vi "Save an I32 Image Vector to FITS with Primary and Extension Headers.vi"(4 "FITS info":T4={"File name"="lsob_demo_0530_LM_20190529_124525_live_C1_00020_001_lev0.0.fits", "Date"="2019-05-29T12:45:25"}, 5 "Andor":T1={"Handle"=0, "Pixel Encoding"="", "AOI Width"=0, "AOI Height"=0, "AOI Stride"=0, "Row Readout Time"=0.0, "Frame Readout Time"=0.0, "Interframe Time"=0.0, "Semaphore"=refnum, "SerialNumber"="", "Camera Model"="", "Controller ID"="", "Firmware Version"="", "Shutter"="Global", "BDiv"=1, "Time at Synch"=timestamp(3029526000.379448 s since 1904-01-01), "Idx"=0, "PreAmp"="", "Binning"=enum."1x1", "PixelReadoutRate"="", "Exposure (s)"=0.05, "Image Bytes"=0, "Image Pixels"=0, "SpuriousNoiseFilter"=FALSE, "Overlap"=FALSE, "CycleMode"=""} {"Exposure (s)" format="%^.3g"; "Time at Synch" format="%<%H:%M:%S>T"; "Interframe Time" format="%#_3g"; "Frame Readout Time" format="%_3g"; "Row Readout Time" format="%_3g"}, 6 "byte order (0:big-endian, network order)":T14(ring), 7 "SCD FITS Cluster":T5={"Wavelength (nm)"=530.15, "Exposure (s)"=0.05, "Tuning Delay (ms)"=1000.0, "Beam Type (-1/1)"=1.0, "Tuning Voltages"=[1.111, 2.222, 3.333, 4.444], "Observer"="observer", "Light Shapping Diffuser"=enum."In Beam", "Comment"="", "Data Type"=9, "Mod Cycles"=0, "SCD Calibration Optics"=enum."1 - Polarizer @0, I+Q", "SCD Emission Line Filter"=enum."1-557.6nm", "Cookbook"="", "COMP-S Calibration Wheel"=enum."Dark", "COMP-S Andover Filter Wheel"=enum."530.3nm/HWB 0.34nm (Fe XIV)", "FOV Rotation (deg)"=66.0, "Objective Lens Position (mm)"=0.0, "Occulter size"=0.0, "Time End"=timestamp(3382374145.421875 s since 1904-01-01), "Acc Exposure (s)"=0.0, "Time Stamp Array"=[], "Camera Serial Number"=[], "Camera Temp"=[], "Camera PI (mm)"=[], "Time Start"=timestamp(3382374145.421875 s since 1904-01-01), "Peripherals"={"ILX controler"=FALSE, "Zone temperatures"=FALSE, "Andor"=FALSE, "Andor 2"=FALSE, "PI Stages"=FALSE, "AISAS mechanisms"=FALSE, "AISAS Mech.lvclass"=refnum, "Zone temp ref"=variant, "FWs"=FALSE}, "FITS paths"=[], "Cameras"=enum."Andor", "load preset cbk"=FALSE, "periodic check count"=0} {"Camera PI (mm)" format="%_3g"; "Acc Exposure (s)" format="%^.3g"; "Occulter size" format="%.2f"; "Objective Lens Position (mm)" min=70.0 max=152.0 format="%.2f"; "FOV Rotation (deg)" format="%.1f"; "Data Type" items=["LIVE", "DARK", "FLAT", "CALI", "OBSE", "ABSO", "AURE", "TARG", "OBJE", "HOLE", "OREX", "THRO", "CHIP"]; "Exposure (s)" format="%^.3g"; "Wavelength (nm)" format="%_6g"}, 8 "error in":errorcluster, 9 "Image Data":u32[](array[numeric]), 10 "Image #":i32=1, 11 "FITS File Path":path=path "G:/SCD Data/Level-0/20160930/20160930T203514.fits") -> (0 "error out":errorcluster, 2 "23040 Byte Header":string="SIMPLE  =                              T / CONFORMS TO FITS STANDARD            BITPIX  =                             32 / BITS PER PIXEL                       NAXIS   =                              2 / DATA DIMENSIONS IN FITS FILE         NAXIS1  =                              0 / XDIM (PIXELS)                        NAXIS2  =                              0 / YDIM (PIXELS)                        NAXIS3  =                              4 / 4 POLARIZATION STATES                NAXIS4  =                              1 / 1 CAMERA                             ORIGIN  =                        'AISAS' / SCIENTIFIC GROUP                     OBSERVER=                     'SCHWARTZ' / NAME OF OBSERVER                     TELESCOP=                   '20CM ZEISS' / NAME OF TELESCOPE                    LOCATION=            'LOMNICKY PEAK OBS' / LOCATION OF TELESCOPE                INSTRUME=                          'SCD' / NAME OF INSTRUMENT                   BZERO   =                             0. /  ADU OFFSET                          FOCUS   =                             26 / CAMERA-STAGE POSITION (MM)           ROTPOS  =                           66.0 / ROTATIONAL POSITION (DEG)            DIFFUSER=                      'IN BEAM' / 0=IN BEAM, 1=OUT OF BEAM             FW-WVLNG=                        '557.6' / PRE-FILTER CENTER WAVELENGTH (NM)    FW-CALIB=                         'DARK' / CAL-WHEEL POSITION                   CAM-SN1 =                    'SCC-02209' / CAMERA SERIAL NUMBER                 CAM-TEMP=                       0.000000 / FOCAL PLANE TEMP (C)                 TUNEDLAY=                           1000 / LCVR RELAXATION DELAY (mS)           DATE_OBS=                     '3/7/2011' / DATE OF OBSERVATION START (UTC)      TIME_OBS=                   '212225.421' / TIME OF OBSERVATION (UTC)            EXPOSURE=                       0.050000 / EXPOSURE TIME (S)                    MODC    =                              0 / NUMBER OF IMAGES AT EACH STATE       NLC-1   =                          1.111 / TUNING VOLTAGE-1                     NLC-2   =                          2.222 / TUNING VOLTAGE-2                     NLC-3   =                          3.333 / TUNING VOLTAGE-3                     NLC-4   =                          4.444 / TUNING VOLTAGE-4                     NLC-5   =                          0.000 / TUNING VOLTAGE-5                     BEAM    =                              1 / BEAM (0=ON BAND OR 1=CONTINUUM)      WAVELENG=                         530.15 / WAVELENGTH OF OBS (NM)               COMMHEAD=                             '' / OBSERVER COMMENT                     COOKBOOK=                                / COOKBOOK  LOADED                     COMMENT                                                                         COMMENT                                                                         COMMENT                                                                         COMMENT                                                                         COMMENT                                                                         COMMENT                                                                         COMMENT                                                                         COMMENT                                                                         COMMENT                                                                         COMMENT                                                                         COMMENT                                                                         COMMENT                                                                         COMMENT                                                                         COMMENT                                                                         COMMENT                                                                         COMMENT                                                                         COMMENT                                                                         COMMENT                                                                         COMMENT                                                                         COMMENT                                                                         COMMENT                                                                         COMMENT                                                                         COMMENT                                                                         COMMENT                                                                         COMMENT                                                                         COMMENT                                                                         COMMENT                                                                         COMMENT                                                                         COMMENT                                                                         COMMENT                                                                         COMMENT                                                                         COMMENT                                                                         COMMENT                                                                         COMMENT                                                                         COMMENT                                                                         COMMENT                                                                         COMMENT                                                                         COMMENT                                                                         COMMENT                                                                         COMMENT                                                                         COMMENT                                                                         COMMENT                                                                         COMMENT                                                                         COMMENT                                                                         COMMENT                                                                         COMMENT                                                                         COMMENT                                                                         COMMENT                                                                         COMMENT                                                                         COMMENT                                                                         COMMENT                                                                         COMMENT                                                                         COMMENT                                                                         COMMENT                                                                         COMMENT                                                                         COMMENT                                                                         COMMENT                                                                         COMMENT                                                                         COMMENT                                                                         COMMENT                                                                         COMMENT                                                                         COMMENT                                                                         COMMENT                                                                         COMMENT                                                                         COMMENT                                                                         COMMENT                                                                         COMMENT                                                                         COMMENT                                                                         COMMENT                                                                         COMMENT                                                                         COMMENT                                                                         COMMENT                                                                         COMMENT                                                                         COMMENT                                                                         COMMENT                                                                         COMMENT                                                                         COMMENT                                                                         COMMENT                                                                         COMMENT                                                                         COMMENT                                                                         COMMENT                                                                         COMMENT                                                                         COMMENT                                                                         COMMENT                                                                         COMMENT                                                                         COMMENT                                                                         COMMENT                                                                         COMMENT                                                                         COMMENT                                                                         COMMENT                                                                         COMMENT                                                                         COMMENT                                                                         COMMENT                                                                         COMMENT                                                                         COMMENT                                                                         COMMENT                                                                         COMMENT                                                                         COMMENT                                                                         COMMENT                                                                         COMMENT                                                                         COMMENT                                                                         COMMENT                                                                         COMMENT                                                                         COMMENT                                                                         COMMENT                                                                         COMMENT                                                                         COMMENT                                                                         COMMENT                                                                         COMMENT                                                                         COMMENT                                                                         COMMENT                                                                         COMMENT                                                                         COMMENT                                                                         COMMENT                                                                         COMMENT                                                                         COMMENT                                                                         COMMENT                                                                         COMMENT                                                                         COMMENT                                                                         COMMENT                                                                         COMMENT                                                                         COMMENT                                                                         COMMENT                                                                         COMMENT                                                                         COMMENT                                                                         COMMENT                                                                         COMMENT                                                                         COMMENT                                                                         COMMENT                                                                         COMMENT                                                                         COMMENT                                                                         COMMENT                                                                         COMMENT                                                                         COMMENT                                                                         COMMENT                                                                         COMMENT                                                                         COMMENT                                                                         COMMENT                                                                         COMMENT                                                                         COMMENT                                                                         COMMENT                                                                         COMMENT                                                                         COMMENT                                                                         COMMENT                                                                         COMMENT                                                                         COMMENT                                                                         COMMENT                                                                         COMMENT                                                                         COMMENT                                                                         COMMENT                                                                         COMMENT                                                                         COMMENT                                                                         COMMENT                                                                         COMMENT                                                                         COMMENT                                                                         COMMENT                                                                         COMMENT                                                                         COMMENT                                                                         COMMENT                                                                         COMMENT                                                                         COMMENT                                                                         COMMENT                                                                         COMMENT                                                                         COMMENT                                                                         COMMENT                                                                         COMMENT                                                                         COMMENT                                                                         COMMENT                                                                         COMMENT                                                                         COMMENT                                                                         COMMENT                                                                         COMMENT                                                                         COMMENT                                                                         COMMENT                                                                         COMMENT                                                                         COMMENT                                                                         COMMENT                                                                         COMMENT                                                                         COMMENT                                                                         COMMENT                                                                         COMMENT                                                                         COMMENT                                                                         COMMENT                                                                         COMMENT                                                                         COMMENT                                                                         COMMENT                                                                         COMMENT                                                                         COMMENT                                                                         COMMENT                                                                         COMMENT                                                                         COMMENT                                                                         COMMENT                                                                         COMMENT                                                                         COMMENT                                                                         COMMENT                                                                         COMMENT                                                                         COMMENT                                                                         COMMENT                                                                         COMMENT                                                                         COMMENT                                                                         COMMENT                                                                         COMMENT                                                                         COMMENT                                                                         COMMENT                                                                         COMMENT                                                                         COMMENT                                                                         COMMENT                                                                         COMMENT                                                                         COMMENT                                                                         COMMENT                                                                         COMMENT                                                                         COMMENT                                                                         COMMENT                                                                         COMMENT                                                                         COMMENT                                                                         COMMENT                                                                         COMMENT                                                                         COMMENT                                                                         COMMENT                                                                         COMMENT                                                                         COMMENT                                                                         COMMENT                                                                         COMMENT                                                                         COMMENT                                                                         COMMENT                                                                         COMMENT                                                                         COMMENT                                                                         COMMENT                                                                         COMMENT                                                                         COMMENT                                                                         COMMENT                                                                         COMMENT                                                                         COMMENT                                                                         COMMENT                                                                         COMMENT                                                                         COMMENT                                                                         COMMENT                                                                         COMMENT                                                                         COMMENT                                                                         COMMENT                                                                         COMMENT                                                                         COMMENT                                                                         COMMENT                                                                         COMMENT                                                                         COMMENT                                                                         COMMENT                                                                         COMMENT                                                                         COMMENT                                                                         COMMENT                                                                         COMMENT                                                                         COMMENT                                                                         COMMENT                                                                         COMMENT                                                                         END                                                                             ", 3 "FITS Path Out":path=path "G:/SCD Data/Level-0/20160930/20160930T203514.fits")   [LabVIEW 2014]
doc: "Duplicate first measurement\nand put it in first element of\nmeasurement array. This\nis a dummy measurement for the\nprimary header. This is because\nwe don't want any images associated\nwith the primary HDU, just the \nextensions. In the Make FITS\nHeaders VI, the NAXIS is set to 0 in\nthis primary HDU"
uses:
  Controls/SCD - FITS Cluster.ctl
  AISAS/Mech/AISAS Mech.lvclass
  AISAS/Controls/Diffuser.ctl
  Controls/SCD - Calibration Optics Filter Wheel.ctl
  Controls/SCD - EDT - Emission Line Filter Wheel.ctl
  Controls/CoMP-S Controls/Polarization Optics Filter Wheel.ctl
  Controls/CoMP-S Controls/Emission Line Filter Wheel.ctl
  AISAS/Controls/focus.ctl
  Controls/peripherals.ctl
  Controls/Cameras select.ctl
  Controls/Fits info.ctl
  Camera/Andor Neo Info.ctl
  Controls/beaning.ctl
  Controls/Globals.vi
panel:
  out "NAXIS":string
  out "# Images in Vector":i32=4
  out "Length of Vector":i32=22118400
  out "Total Pixels":i64=5529600
  out "AOI Height":i64=2160
  out "AOI Width":i64=2560
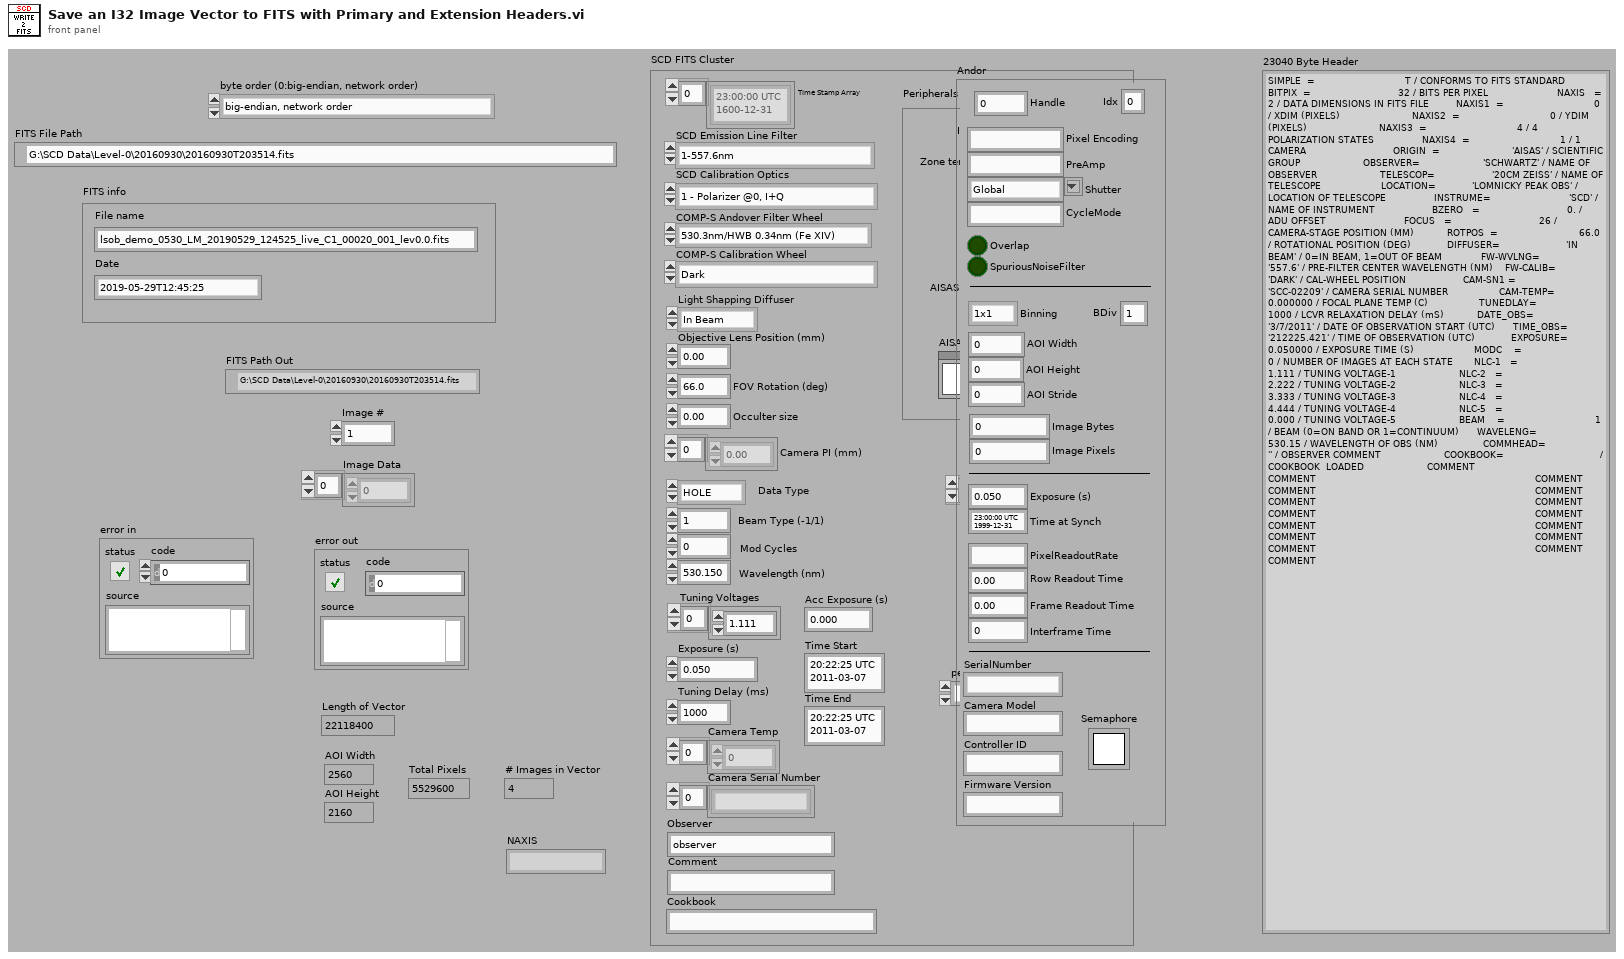
[diagram p1: front panel]
types:
  T1 = typedef "Andor Neo Info.ctl" = cluster{"Handle":i32, "Pixel Encoding":string, "AOI Width":i32, "AOI Height":i32, "AOI Stride":i32, "Row Readout Time":dbl, "Frame Readout Time":dbl, "Interframe Time":dbl, "Semaphore":T2, "SerialNumber":string, "Camera Model":string, "Controller ID":string, "Firmware Version":string, "Shutter":string, "BDiv":u8, "Time at Synch":timestamp, "Idx":i32, "PreAmp":string, "Binning":T3, "PixelReadoutRate":string, "Exposure (s)":dbl, "Image Bytes":i64, "Image Pixels":i64, "SpuriousNoiseFilter":bool, "Overlap":bool, "CycleMode":string}
  T2 = typedef "Semaphore RefNum" = refnum<k1>
  T3 = typedef "beaning.ctl" = enum16{"1x1", "2x2", "3x3", "4x4", "8x8"}
  T4 = typedef "Fits info.ctl" = cluster{"File name":string, "Date":string}
  T5 = typedef "SCD - FITS Cluster.ctl" = cluster{"Wavelength (nm)":dbl, "Exposure (s)":dbl, "Tuning Delay (ms)":dbl, "Beam Type (-1/1)":dbl, "Tuning Voltages":dbl[], "Observer":string, "Light Shapping Diffuser":T6, "Comment":string, "Data Type":u16, "Mod Cycles":u16, "SCD Calibration Optics":T7, "SCD Emission Line Filter":T8, "Cookbook":string, "COMP-S Calibration Wheel":T9, "COMP-S Andover Filter Wheel":T10, "FOV Rotation (deg)":dbl, "Objective Lens Position (mm)":T11, "Occulter size":dbl, "Time End":timestamp, "Acc Exposure (s)":dbl, "Time Stamp Array":timestamp[], "Camera Serial Number":string[], "Camera Temp":dbl[], "Camera PI (mm)":dbl[], "Time Start":timestamp, "Peripherals":T12, "FITS paths":path[], "Cameras":T13, "load preset cbk":bool, "periodic check count":i32}
  T6 = typedef "Diffuser.ctl" = enum16{"Out of Beam", "In Beam"}
  T7 = typedef "SCD - Calibration Optics Filter Wheel.ctl" = enum16{"1 - Polarizer @0, I+Q", "2 - Polarizer @90, I-Q", "3 - Polarizer @45, I+U", "4 - Polarizer @135, I-U", "5 - Polarizer @0, Retarder @45, I+V", "6 - Polarizer @0, Retarder @135, I-V", "7 - Dark", "8 - Clear", "9 - N/A"}
  T8 = typedef "SCD - EDT - Emission Line Filter Wheel.ctl" = enum16{"1-557.6nm", "2-587.6nm", "3-589.6nm", "4-630.2nm", "5-656.4nm", "6-849.8nm", "7-854.2nm", "8-866.2nm", "9-1083.0nm"}
  T9 = typedef "Polarization Optics Filter Wheel.ctl" = enum16{"Dark", "Clear", "Exchange Lens", "Polarizer @0, I+Q", "Polarizer @90, I-Q", "Polarizer @45, I+U", "Polarizer @135, I-U", "Polarizer @0, Retarder @45, I+V", "Polarizer @0, Retarder @135, I-V"}
  T10 = typedef "Emission Line Filter Wheel.ctl" = enum16{"530.3nm/HWB 0.34nm (Fe XIV)", "587.6nm/HBW 0.44nm (He I D3)", "637.5nm/HBW 0.53nm (Fe X)", "656.3nm/HBW 0.57nm (H-Alpha)", "789.2nm/HBW 0.85nm (Fe XI)", "854.2nm/HBW 1.01nm (Ca I)", "1074.7nm/HBW 2.34nm (Fe XIII)", "1079.8nm/HBW 1.64nm (Fe XIII)", "1083.0nm/HBW 1.66nm (He I)"}
  T11 = typedef "focus.ctl" = dbl
  T12 = typedef "peripherals.ctl" = cluster{"ILX controler":bool, "Zone temperatures":bool, "Andor":bool, "Andor 2":bool, "PI Stages":bool, "AISAS mechanisms":bool, "AISAS Mech.lvclass":refnum<class "AISAS Mech.lvclass">, "Zone temp ref":variant, "FWs":bool}
  T13 = typedef "Cameras select.ctl" = enum16{"Andor", "GDR"}
  T14 = enum16{"big-endian, network order", "native, host order", "little-endian"}
  T15 = enum16{"open", "replace", "create", "open or create", "replace or create", "replace or create with confirmation"}
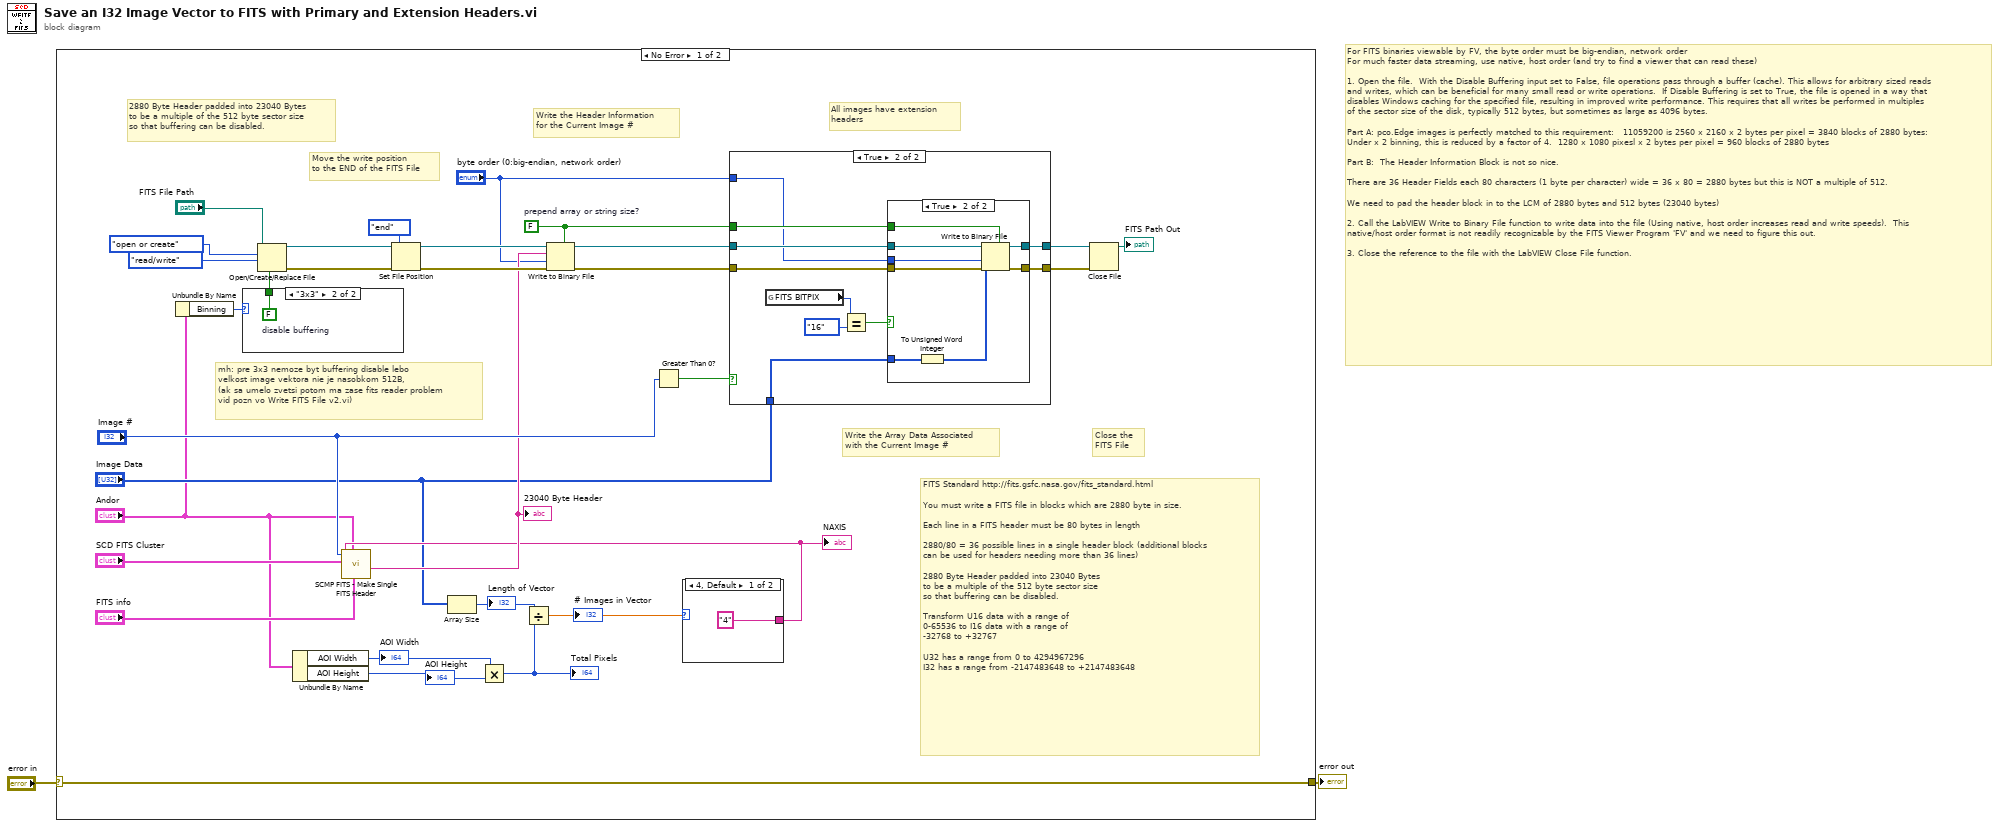
[diagram p0: block diagram]
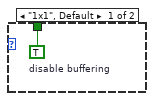
[diagram p2: hidden frame]
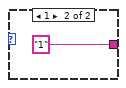
[diagram p3: hidden frame]
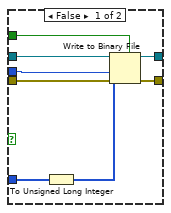
[diagram p5: hidden frame]
diagram:
  # "For FITS binaries viewable by FV, the byte order must be big-endian, network order\nFor much faster data streaming, use native, host order (and try to find a viewer that can read these)\n\n1. Open the file.  With the Disable Buffering input set to False, file operations pass through a buffer (cache). This allows for arbitrary sized reads and writes, which can be beneficial for many small read or write operations.  If Disable Buffering is set to True, the file is opened in a way that disables Windows caching for the specified file, resulting in improved write performance. This requires that all writes be performed in multiples of the sector size of the disk, typically 512 bytes, but sometimes as large as 4096 bytes.\n\nPart A: pco.Edge images is perfectly matched to this requirement:   11059200 is 2560 x 2160 x 2 bytes per pixel = 3840 blocks of 2880 bytes:  Under x 2 binning, this is reduced by a factor of 4.  1280 x 1080 pixesl x 2 bytes per pixel = 960 blocks of 2880 bytes\n\nPart B:  The Header Information Block is not so nice.  \n\nThere are 36 Header Fields each 80 characters (1 byte per character) wide = 36 x 80 = 2880 bytes but this is NOT a multiple of 512.\n\nWe need to pad the header block in to the LCM of 2880 bytes and 512 bytes (23040 bytes)\n\n2. Call the LabVIEW Write to Binary File function to write data into the file (Using native, host order increases read and write speeds).  This native/host order format is not readily recognizable by the FITS Viewer Program 'FV' and we need to figure this out.\n\n3. Close the reference to the file with the LabVIEW Close File function."
  n1 = case shown="No Error" "error in" {
    selector: "error in" -> [w27 w66]
    tunnel: [w27 w66] -> w1
    frame No Error {
      w24 = FALSE  # prepend array or string size?
      # "mh: pre 3x3 nemoze byt buffering disable lebo\nvelkost image vektora nie je nasobkom 512B,\n(ak sa umelo zvetsi potom ma zase fits reader problem\nvid pozn vo Write FITS File v2.vi)"
      # "All images have extension \nheaders"
      # "2880 Byte Header padded into 23040 Bytes\nto be a multiple of the 512 byte sector size\nso that buffering can be disabled."
      # "FITS Standard http://fits.gsfc.nasa.gov/fits_standard.html\n\nYou must write a FITS file in blocks which are 2880 byte in size.\n\nEach line in a FITS header must be 80 bytes in length\n\n2880/80 = 36 possible lines in a single header block (additional blocks\ncan be used for headers needing more than 36 lines)\n\n2880 Byte Header padded into 23040 Bytes\nto be a multiple of the 512 byte sector size\nso that buffering can be disabled.\n\nTransform U16 data with a range of\n0-65536 to I16 data with a range of\n-32768 to +32767\n\nU32 has a range from 0 to 4294967296\nI32 has a range from -2147483648 to +2147483648"
      # "Close the \nFITS File"
      # "Write the Array Data Associated\nwith the Current Image #"
      # "Write the Header Information\nfor the Current Image #"
      # "Move the write position\nto the END of the FITS File"
      n2 = Unbundle By Name("Andor") -> ("Binning"=w3:T3)
      n3 = case shown="\"3x3\"" w3 {
        tunnel: [w34 w35] -> w28
        frame "1x1", Default {
          w34 = TRUE  # disable buffering
        }
        frame "3x3" {
          w35 = FALSE  # disable buffering
        }
      }
      n4 = Open/Create/Replace File(file path (use dialog)="FITS File Path", operation (0:open)=T15."open or create", access (0:read/write)=enum16{"read/write", "read-only", "write-only"}."read/write", disable buffering (F)=w28) -> (refnum out=w20:refnum<file>, error out=w21:errorcluster)  [unwired: 1 in, 2 out]
      n5 = Unbundle By Name("Andor") -> ("AOI Width"=w15:i32, "AOI Height"=w16:i32)
      "AOI Width" <- w15
      "AOI Height" <- w16
      n6 = Set File Position(refnum=w20, from (0:start)=enum16{"start", "end", "current"}."end" ("pos mode (0:2)"), error in=w21) -> (refnum out=w19:refnum<file>, error out=w18:errorcluster)  [unwired: 1 out]
      n7 = Array Size(array="Image Data") -> (size(s)=w14:i32)
      "Length of Vector" <- w14
      n8 = Multiply(x=w15, y=w16) -> (x*y=w13:i32)
      "Total Pixels" <- w13
      n9 = Divide(x=w14, y=w13) -> (x/y=w10:dbl)
      "# Images in Vector" <- w10
      n10 = Greater Than 0?(x="Image #") -> (x > 0?=w23:bool)
      n11 = case shown="4, Default" w10 {
        tunnel: ["4" ("NAXIS") "1" ("NAXIS")] -> w9
        frame 4, Default {
        }
        frame 1 {
        }
      }
      "NAXIS" <- w9
      n12 = call "SCMP FITS - Make Single FITS Header.vi"("FITS info"="FITS info", "Andor"="Andor", "NAXIS"=w9, "FITS Header"="SCD FITS Cluster", "Image #"="Image #") -> ("23040 Byte Header"=w11:string)  [unwired: 1 in, 5 out]
      "23040 Byte Header" <- w11
      n13 = Write to Binary File(file (use dialog)=w19, data=w11, error in=w18, 5:w24, 9:"byte order (0:big-endian, network order)") -> (refnum out=w25:refnum<file>, error out=w26:errorcluster)  [unwired: 2 out]
      n14 = case shown="True" w23 {
        tunnel: [w38 w49] -> w33
        tunnel: [w39 w48] -> w32
        tunnel: w26 -> [w38 w45]
        tunnel: w25 -> [w39 w46]
        tunnel: w24 -> [_ w47]
        tunnel: "Image Data" -> [_ w44]
        tunnel: "byte order (0:big-endian, network order)" -> [_ w40]
        frame False {
          # "Primary Headers have no associated image.  \nAll we've done so far is to create a blank FITS \nfile and write a Primary Header"
        }
        frame True {
          n15 = global read "Globals.vi" "FITS BITPIX"() -> (w42:enum16{"16", "32"})
          n16 = Equal?(x=w42, y=enum16{"16", "32"}."16") -> (x = y?=w41:bool)
          n17 = case shown="True" w41 {
            tunnel: [w51 w65] -> w49
            tunnel: [w50 w64] -> w48
            tunnel: w47 -> [w54 w63]
            tunnel: w46 -> [w55 w62]
            tunnel: w45 -> [w56 w61]
            tunnel: w44 -> [w53 w60]
            tunnel: w40 -> [w52 w58]
            frame False {
              n18 = To Unsigned Long Integer(number=w53) -> (unsigned 32bit integer=w57:u32[])
              n19 = Write to Binary File(file (use dialog)=w55, data=w57, error in=w56, 5:w54, 9:w52) -> (refnum out=w50:refnum<file>, error out=w51:errorcluster)  [unwired: 2 out]
            }
            frame True {
              n20 = To Unsigned Word Integer(number=w60) -> (unsigned 16bit integer=w59:u16[])
              n21 = Write to Binary File(file (use dialog)=w62, data=w59, error in=w61, 5:w63, 9:w58) -> (refnum out=w64:refnum<file>, error out=w65:errorcluster)  [unwired: 2 out]
            }
          }
        }
      }
      n22 = Close File(refnum=w32, error in=w33) -> (path=→"FITS Path Out":path)  [unwired: 1 out]
    }
    frame Error {
    }
  }
  "error out" <- w1
